vi "Main_SubVI_Motion Status.vi"(8 "Error In":errorcluster, 11 "Normal Array In":string[](array[string])) -> (0 "Error Out":errorcluster, 2 "Response":string, 3 "Status":T1)   [LabVIEW 2015]
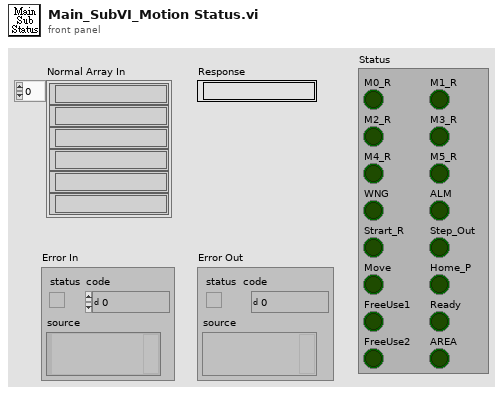
[diagram p1: front panel]
types:
  T1 = cluster{"M0_R":bool, "M1_R":bool, "M2_R":bool, "M3_R":bool, "M4_R":bool, "M5_R":bool, "WNG":bool, "ALM":bool, "Strart_R":bool, "Step_Out":bool, "Move":bool, "Home_P":bool, "FreeUse1":bool, "Ready":bool, "FreeUse2":bool, "AREA":bool}
  T2 = cluster{"Boolean array[0]":bool, "Boolean array[1]":bool, "Boolean array[2]":bool, "Boolean array[3]":bool, "Boolean array[4]":bool, "Boolean array[5]":bool, "Boolean array[6]":bool, "Boolean array[7]":bool, "Boolean array[8]":bool, "Boolean array[9]":bool, "Boolean array[10]":bool, "Boolean array[11]":bool, "Boolean array[12]":bool, "Boolean array[13]":bool, "Boolean array[14]":bool, "Boolean array[15]":bool}
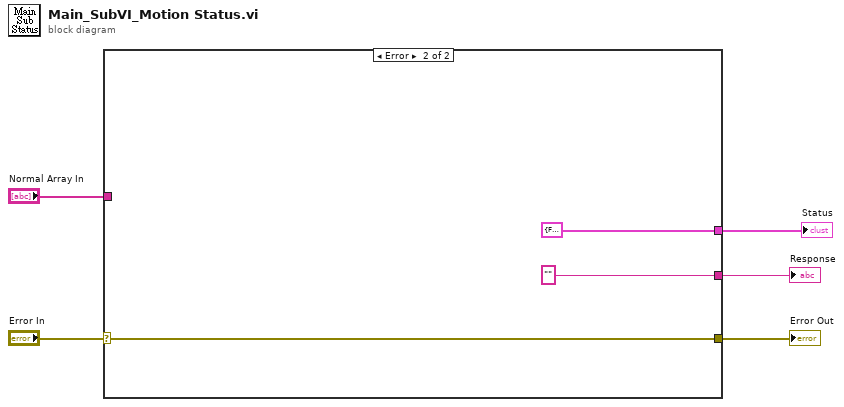
[diagram p0: block diagram]
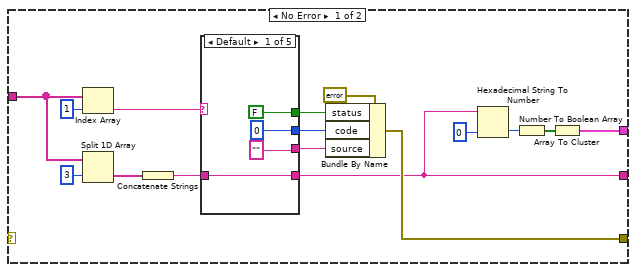
[diagram p2: hidden frame]
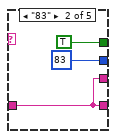
[diagram p3: hidden frame]
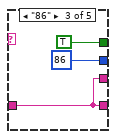
[diagram p4: hidden frame]
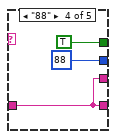
[diagram p5: hidden frame]
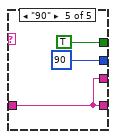
[diagram p6: hidden frame]
diagram:
  n1 = case shown="Error" "Error In" {
    selector: "Error In" -> [_ w40]
    tunnel: "Normal Array In" -> [w13 _]
    tunnel: [w11 w40] -> w3
    tunnel: [w7 ""] -> w2
    tunnel: [w6 T2 {"Boolean array[0]"=FALSE, "Boolean array[1]"=FALSE, "Boolean array[2]"=FALSE, "Boolean array[3]"=FALSE, "Boolean array[4]"=FALSE, "Boolean array[5]"=FALSE, "Boolean array[6]"=FALSE, "Boolean array[7]"=FALSE, "Boolean array[8]"=FALSE, "Boolean array[9]"=FALSE, "Boolean array[10]"=FALSE, "Boolean array[11]"=FALSE, "Boolean array[12]"=FALSE, "Boolean array[13]"=FALSE, "Boolean array[14]"=FALSE, "Boolean array[15]"=FALSE} ("Boolean array")] -> w1
    frame No Error {
      n2 = Index Array(array=w13, index=1) -> (element=w21:string)
      n3 = Split 1D Array(array=w13, index=3) -> (second subarray=w19:string[])  [unwired: 1 out]
      n4 = Concatenate Strings(w19) -> (w18:string)
      n5 = case shown="Default" w21 {
        tunnel: w18 -> [w23 w26 w29 w33 w35]
        tunnel: [w23 w26 w29 w33 w35] -> w7
        tunnel: [FALSE TRUE TRUE TRUE TRUE] -> w16
        tunnel: [0 ("code") 83 ("code") 86 ("code") 88 ("code") 90 ("code")] -> w15
        tunnel: ["" w26 w29 w33 w35] -> w14
        frame Default {
        }
        frame "83" {
        }
        frame "86" {
        }
        frame "88" {
        }
        frame "90" {
        }
      }
      n6 = Bundle By Name(cluster=errorcluster {"status"=FALSE, "code"=0, "source"=""} ("error constant"), "status"=w16, "code"=w15, "source"=w14) -> (w11:errorcluster)
      n7 = Hexadecimal String To Number(string=w7, default (0uL)=0 ("default (0 U32)")) -> (number=w9:i32)  [unwired: 1 in, 1 out]
      n8 = Number To Boolean Array(number=w9) -> (Boolean array=w10:bool[])
      n9 = Array To Cluster(array=w10) -> (cluster=w6:T2)
    }
    frame Error {
    }
  }
  "Error Out" <- w3
  "Response" <- w2
  "Status" <- w1
